vi "GetNI_SynthFoc.vi"(0 "Digitizer Settings":T4={"Digitizer delay (us) "=0.0, "rf points per line"=2048, "lines per plane"=128, "Samp Rate (Hz)"=100000000.0, "Additional dig delay (us)"=0.0, "Voltage Scale"=0.4, "Pre-Looks"=0, "Offset delay (us)"=0.0, "bits A/D"=8, "Avg Num"=1, "DigTimeOut"=5.0, "Rel Dig Delay"=0.0, "Dig Ch"=0, "LeCroyCluster"={"LeCroy Channels"=[TRUE, FALSE, FALSE, FALSE], "LC read pt offset"=0.0, "Sweep Avg"=FALSE}, "Main Digitizer"=enum."NI Digitizer", "Dig Config"=enum."Single channel", "Digitizer ID Cluster"={"Acqiris/Alazar/SP ID"=[], "NI Instr Handles"=[], "LeCroy VISA"="", "GaGe Handle"={"Handle"=0, "Sample size"=0, "Resolution"=0, "Offset"=0, "Channels"=0, "Boards"=0}, "ATS Ref"="ATS9350", "Acqiris Address"=["PCI::INSTR0"], "ADQRef"=refnum, "adq_cu_ptr"=refnum}, "Trigger Settings"={"Trig Source"=1, "Trig Coupling"=0, "Trig Slope"=0, "Level (mV)"=1500.0}, "Bulk Acq"=FALSE, "Bulk Start Indexes"=[], "Data Ref RF"=refnum, "NI ID/Channel"=[], "Total Dig CH"=1, "Xtra Ann Trig delay (us)"=10.0, "Fix Z Delay?"=FALSE, "One Way Transmission?"=FALSE, "Data Ref Log"=refnum} {"Trigger Settings"."Trig Slope" items=["Positive", "Negative"]; "Trigger Settings"."Level (mV)" format="%.2f"; "Trigger Settings"."Trig Coupling" items=["DC 1 MOhm", "AC 1 MOhm", "DC 50 Ohm", "AC 50 Ohm"]; "Trigger Settings"."Trig Source" items=["Chan 1", "External"]; "Rel Dig Delay" format="%.2f"; "DigTimeOut" format="%.2f"; "Avg Num" min=1; "Offset delay (us)" format="%.2f"; "Additional dig delay (us)" format="%.2f"; "Digitizer delay (us)" format="%.2f"}, 3 "NI Card":refnum<k15>, 5 "Ann Array Params":T1={"Synth Foc?"=FALSE, "Focal Zones"=41, "Switch T/R"=0, "Trans Geometry (mm)"={"Transducer"=0, "Geo Focus"=12.0, "a (radius)"=3.0, "# of rings"=5, "kerf space "=0.1, "Center Freq"=12.0}, "Sub Ap Excite?"=FALSE, "Full Array Scan?"=FALSE, "Xmt/Rcv"={"XMIT"=[TRUE, TRUE, TRUE, TRUE, TRUE], "RCV"=[TRUE, TRUE, TRUE, TRUE, TRUE]}, "PulseSpacing (us)"=0.0, "Xmit Ring"=0, "XMIT CHS"=0, "RCV CHS"=0, "GPU?"=FALSE, "Save TIFF?"=FALSE, "downfactor"=1, "RCV 1CH"=0} {"RCV 1CH" items=["All", "1", "2", "3", "4", "5"]; "Trans Geometry (mm)"."Transducer" items=["6D 12R 40 MHz"=0, "10D 31R 20 MHz"=1, "10D 23R 20 MHz"=2, "6D 23R 40 MHz"=3, "4.5D 10.7R 40 MHz"=4, "9D 23.5R 20 MHz"=5, "9D 25.8R 20MHz"=6, "Enter"=99]; "Switch T/R" min=1 max=5 step=1}, 7 "errorin":errorcluster, 8 "File Array":string[](array[string]), 11 "Reverse ?":bool, 13 "Rcv Ring":i32) -> (17 "Raw VGain (scale)":dbl, 18 "Gain Array":T8(array[cluster]), 21 "VGain (dB)":dbl, 25 "Synth App Out":i16[][](array[numeric]), 27 "error out":errorcluster)   [LabVIEW 2022 SP3]
uses:
  -DigitizerRoutines/DigitizerSettings.ctl
  -DigitizerRoutines/Digitizer.ctl
  -DigitizerRoutines/DigConfig.ctl
  -DigitizerRoutines/DigitizerID.ctl
  C:/Windows/System32/ADQAPI_dotNet_helper.dll
  Annular Array/-AnnularRoutines/AnnularArray.ctl
  Annular Array/-AnnularRoutines/TransGeometry.ctl
  Annular Array/-AnnularRoutines/ArrayGeometry.ctl
  <instrlib>/niScope/Acquire/Fetch/niScope Multi Fetch Binary 8.vi
  Annular Array/-SynthApperture/ProcImageHD_I8.vi
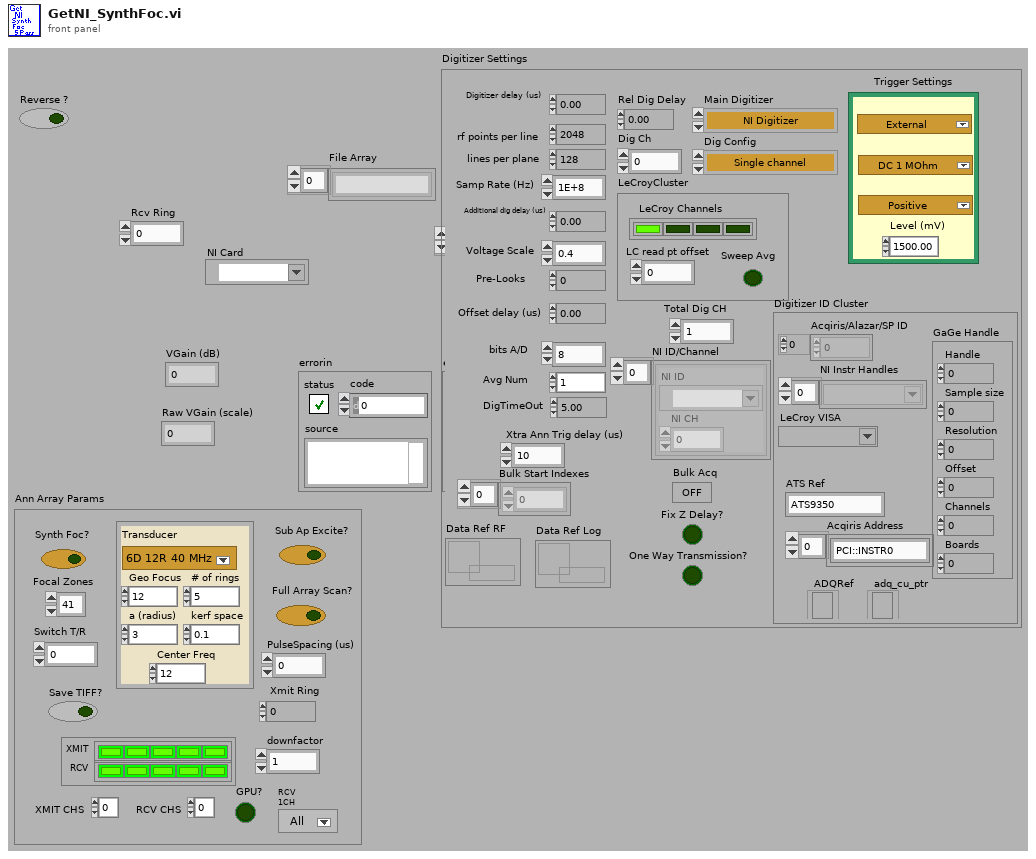
[diagram p1: front panel]
types:
  T1 = typedef "AnnularArray.ctl" = cluster{"Synth Foc?":bool, "Focal Zones":i16, "Switch T/R":i16, "Trans Geometry (mm)":T2, "Sub Ap Excite?":bool, "Full Array Scan?":bool, "Xmt/Rcv":cluster{"XMIT":bool[], "RCV":bool[]}, "PulseSpacing (us)":sgl, "Xmit Ring":i32, "XMIT CHS":u8, "RCV CHS":u8, "GPU?":bool, "Save TIFF?":bool, "downfactor":i32, "RCV 1CH":u16}
  T2 = typedef "TransGeometry.ctl" = cluster{"Transducer":T3, "Geo Focus":dbl, "a (radius)":dbl, "# of rings":i32, "kerf space ":dbl, "Center Freq":dbl}
  T3 = typedef "ArrayGeometry.ctl" = u16
  T4 = typedef "DigitizerSettings.ctl" = cluster{"Digitizer delay (us) ":dbl, "rf points per line":i32, "lines per plane":i32, "Samp Rate (Hz)":dbl, "Additional dig delay (us)":dbl, "Voltage Scale":dbl, "Pre-Looks":i32, "Offset delay (us)":dbl, "bits A/D":i8, "Avg Num":i32, "DigTimeOut":sgl, "Rel Dig Delay":sgl, "Dig Ch":i32, "LeCroyCluster":cluster{"LeCroy Channels":bool[], "LC read pt offset":dbl, "Sweep Avg":bool}, "Main Digitizer":T5, "Dig Config":T6, "Digitizer ID Cluster":T7, "Trigger Settings":cluster{"Trig Source":u16, "Trig Coupling":u16, "Trig Slope":u16, "Level (mV)":dbl}, "Bulk Acq":bool, "Bulk Start Indexes":i32[], "Data Ref RF":refnum<data-value>, "NI ID/Channel":cluster{"NI ID":refnum<k15>, "NI CH":i32}[], "Total Dig CH":i32, "Xtra Ann Trig delay (us)":dbl, "Fix Z Delay?":bool, "One Way Transmission?":bool, "Data Ref Log":refnum<data-value>}
  T5 = typedef "Digitizer.ctl" = enum16{"Acqiris Digitizer", "NI Digitizer", "LeCroy", "GaGe", "AlazarTech", "No Digitizer", "Teledyne"}
  T6 = typedef "DigConfig.ctl" = enum16{"Single channel", "2 Chans w/ 2 Acqiris", "2 Chans w/ 1 Acqiris", "5-CH Pulser New", "5-CH pulser w/ ann array", "5-pass style ann array", "Empty"}
  T7 = typedef "DigitizerID.ctl" = cluster{"Acqiris/Alazar/SP ID":u32[], "NI Instr Handles":refnum<k15>[], "LeCroy VISA":refnum<visa-resource-name>, "GaGe Handle":cluster{"Handle":u32, "Sample size":u32, "Resolution":i32, "Offset":i32, "Channels":u32, "Boards":u32}, "ATS Ref":string, "Acqiris Address":string[], "ADQRef":refnum<k24>, "adq_cu_ptr":refnum<k24>}
  T8 = cluster{sgl, "Gain [dB]  ":sgl, "Atten (dB)":sgl}[]
  T9 = cluster{"actualSamples":i32, "absoluteInitialX":dbl, "relativeInitialX":dbl, "xIncrement":dbl, "offset":dbl, "gain":dbl, "reserved1":dbl, "reserved2":dbl}[]
  T10 = cluster{"actualSamples":i32, "absoluteInitialX":dbl, "relativeInitialX":dbl, "xIncrement":dbl, "offset":dbl, "gain":dbl, "reserved1":dbl, "reserved2":dbl}
  T11 = cluster{sgl, "Gain [dB]  ":sgl, "Atten (dB)":sgl}
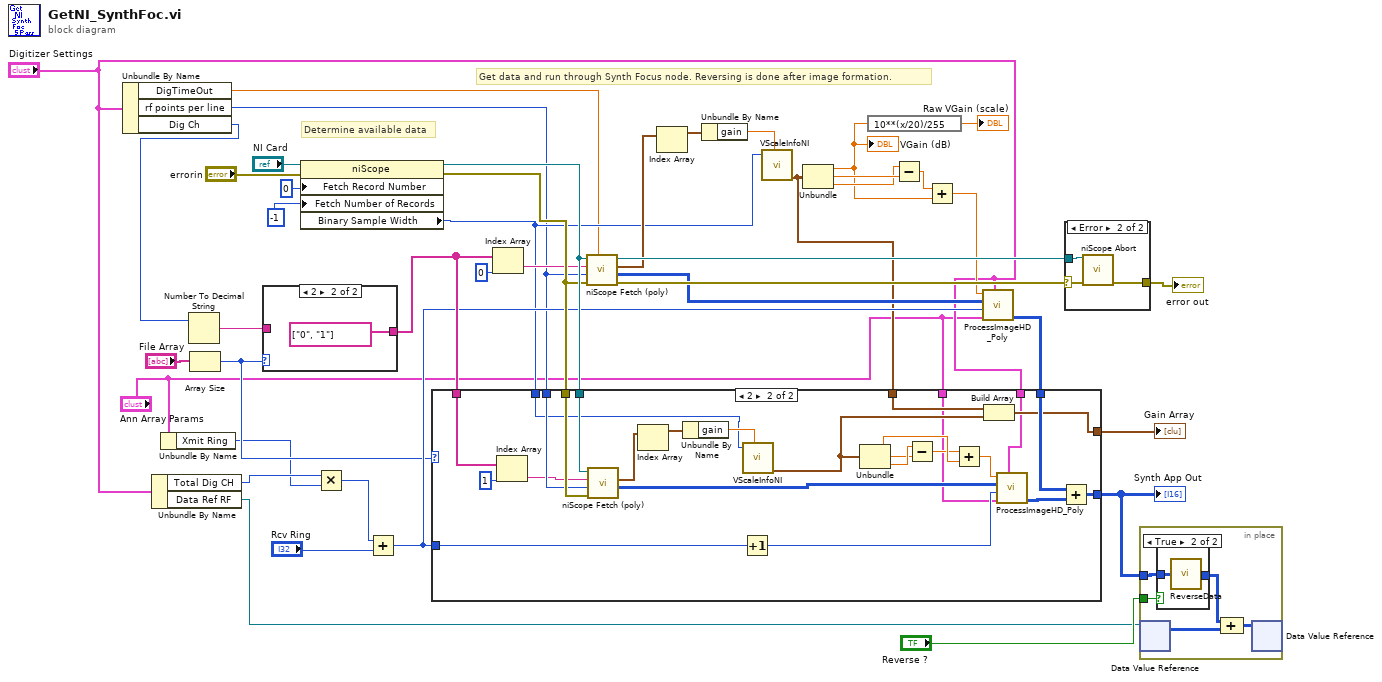
[diagram p0: block diagram]
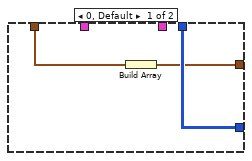
[diagram p3: hidden frame]
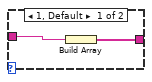
[diagram p4: hidden frame]
diagram:
  # "Get data and run through Synth Focus node. Reversing is done after image formation."
  # "Determine available data"
  n1 = Unbundle By Name("Digitizer Settings") -> ("DigTimeOut"=w10:sgl, "rf points per line"=w11:i32, "Dig Ch"=w9:i32)
  n2 = Unbundle By Name("Digitizer Settings") -> ("Total Dig CH"=w7:i32, "Data Ref RF"=w1:refnum<data-value>)
  n3 = Unbundle By Name("Ann Array Params") -> ("Xmit Ring"=w4:i32)
  n4 = Number To Decimal String(number=w9) -> (decimal integer string=w33:string)  [unwired: 1 out]
  n5 = Array Size(array="File Array") -> (size(s)=w17:i32)
  n6 = case shown="2" w17 {
    tunnel: [w44 string[] ["0", "1"] ("File Array")] -> w21
    tunnel: w33 -> [w43 _]
    frame 1, Default {
      n7 = Build Array(w43) -> (w44:string[])
    }
    frame 2 {
    }
  }
  n8 = property class="niScope"(reference="NI Card", error in="errorin", "Fetch Record Number"=0 ("Fetch:Fetch Record Number"), "Fetch Number of Records"=-1 ("Fetch:Fetch Number of Records")) -> (reference out=w25:refnum<k15>, error out=w24:errorcluster, "Binary Sample Width"=w12:i32)
  n9 = Multiply(x=w7, y=w4) -> (x*y=w6:i32)
  n10 = Add(x=w6, y="Rcv Ring") -> (x+y=w19:i32)
  n11 = Index Array(array=w21, index=0) -> (element=w22:string)
  n12 = call-poly <instrlib>:"niScope Fetch (poly).vi"("timeout"=w10, "error in"=w24, "numSamples"=w11, "channels"=w22, "instrument handle"=w25) -> ("error out"=w30:errorcluster, "wfm"=w20:i8[][], "wfm info"=w28:T9, "instrument handle out"=w29:refnum<k15>)  [unwired: 3 out]
  n13 = Index Array(array=w28) -> (element=w27:T10)  [unwired: 1 in]
  n14 = Unbundle By Name(w27) -> ("gain"=w26:dbl)
  n15 = call "VScaleInfoNI.vi"("A/D bits"=w12, "gain"=w26) -> ("Voltage Scale"=w14:T11)  [unwired: 5 in, 3 out]
  n16 = Unbundle(w14) -> (w38:sgl, "Gain [dB]"=w40:sgl, "Atten (dB)"=w39:sgl)
  "VGain (dB)" <- w38
  n17 = expression code="10**(x/20)/255"(w38) -> (→"Raw VGain (scale)":sgl)
  n18 = Subtract(x=w39, y=w40) -> (x-y=w41:sgl)
  n19 = Add(x=w41, y=w38) -> (x+y=w18:sgl)
  n20 = call-poly "ProcessImageHD_Poly.vi"("Digitizer Settings"="Digitizer Settings", "Ann Array Params"="Ann Array Params", "T/R Ring"=w19, "Scan Data In"=w20, "Att (dB)"=w18) -> ("Synth App Out"=w13:i16[][])  [unwired: 3 in, 1 out]
  n21 = case shown="2" w17 {
    tunnel: w25 -> [_ w74]
    tunnel: w24 -> [_ w73]
    tunnel: w11 -> [_ w72]
    tunnel: w21 -> [_ w69]
    tunnel: w19 -> [_ w65]
    tunnel: w13 -> [w48 w64]
    tunnel: [w48 w63] -> w3
    tunnel: [w46 w52] -> w15
    tunnel: w14 -> [w47 w54]
    tunnel: w12 -> [_ w51]
    tunnel: "Digitizer Settings" -> [_ w50]
    tunnel: "Ann Array Params" -> [_ w49]
    frame 0, Default {
      n22 = Build Array(w47) -> (w46:T8)
    }
    frame 2 {
      n23 = Index Array(array=w69, index=1) -> (element=w70:string)
      n24 = call-poly <instrlib>:"niScope Fetch (poly).vi"("error in"=w73, "numSamples"=w72, "channels"=w70, "instrument handle"=w74) -> ("wfm"=w66:i8[][], "wfm info"=w60:T9)  [unwired: 1 in, 5 out]
      n25 = Index Array(array=w60) -> (element=w62:T10)  [unwired: 1 in]
      n26 = Unbundle By Name(w62) -> ("gain"=w61:dbl)
      n27 = Increment(x=w65) -> (x+1=w68:i32)
      n28 = call "VScaleInfoNI.vi"("A/D bits"=w51, "gain"=w61) -> ("Voltage Scale"=w53:T11)  [unwired: 5 in, 3 out]
      n29 = Unbundle(w53) -> (w59:sgl, "Gain [dB]"=w57:sgl, "Atten (dB)"=w58:sgl)
      n30 = Subtract(x=w58, y=w57) -> (x-y=w56:sgl)
      n31 = Add(x=w56, y=w59) -> (x+y=w55:sgl)
      n32 = Build Array(w54, w53) -> (w52:T8)
      n33 = call-poly "ProcessImageHD_Poly.vi"("Digitizer Settings"=w50, "Ann Array Params"=w49, "T/R Ring"=w68, "Scan Data In"=w66, "Att (dB)"=w55) -> ("Synth App Out"=w67:i16[][])  [unwired: 3 in, 1 out]
      n34 = Add(x=w64, y=w67) -> (x+y=w63:i16[][])
    }
  }
  "Gain Array" <- w15
  "Synth App Out" <- w3
  n35 = case shown="Error" w30 {
    selector: w30 -> [w75 w76]
    tunnel: [w75 w78] -> w37
    tunnel: w29 -> [_ w77]
    frame No Error {
    }
    frame Error {
      n36 = call <instrlib>:"niScope Abort.vi"("instrument handle"=w77, "error in"=w76) -> ("error out"=w78:errorcluster)  [unwired: 13 out]
    }
  }
  "error out" <- w37
  n37 = in-place {
    in-place-border: w3 -> [w80]
    in-place-border: "Reverse ?" -> [w79]
    n38 = in-place-dvr #1(w1) -> (w83:i16[][])  [unwired: 1 out]
    n39 = case shown="True" w79 {
      tunnel: w80 -> [w84 w86]
      tunnel: [w84 w85] -> w81
      frame False {
      }
      frame True {
        n40 = call "ReverseData.vi"("Array in"=w86) -> ("Array out"=w85:i16[][])
      }
    }
    n41 = Compound Arithmetic op=ADD(w81, w83) -> (w82:i16[][])
    n42 = in-place-dvr #1(w82) -> ()  [unwired: 2 out]
  }
